vi "rvc SIM Quadcopter.vi"(7 "omega2":dbl, 9 "omega4":dbl, 10 "omega3":dbl, 11 "omega1":dbl) -> (3 "States":dbl[](array[numeric])=[0.0, 0.0, 0.0, 2.3184100418409948, 0.0, 0.0])   [LabVIEW 2013]
uses:
  <vilib>/Simulation/Implementation/Shared/SIMSCR Execution Mode.ctl
  <vilib>/Simulation/Scripting/Companion Diagram/SimConfigNode/SimParams.ctl
  <vilib>/Simulation/Scripting/Companion Diagram/SimConfigNode/_simSolvers.ctl
  <vilib>/Simulation/Param Hierarchy/Typedefs/SIMPH Param Control Actions.ctl
  <vilib>/Simulation/Implementation/Shared/SIM limit type.ctl
  <vilib>/Simulation/Implementation/Shared/NILVSim_ParamChanged.vi
  <vilib>/Simulation/Implementation/Shared/NILVSIM_BeginStep.vi
  <vilib>/Simulation/ContinuousLinear/Implementation/NILVSim Integrator new.llb/SIM Integrator Distributor (vector).vi
  <vilib>/Simulation/ContinuousLinear/Implementation/NILVSim Integrator new.llb/SIM Integrator Collector (vector).vi
  <vilib>/Simulation/Implementation/Shared/NILVSim_Manager.vi
  <vilib>/Simulation/Implementation/Shared/NILVSim_FinalizeModel.vi
  <vilib>/Simulation/Implementation/Shared/SIM Unbundle Sim Info.vi
  <vilib>/Utility/error.llb/Clear Errors.vi
  <vilib>/Simulation/Implementation/Shared/NILVSim_GetModelError.vi
  <vilib>/Simulation/Implementation/Shared/SIM SimErrorHandler.vi
  <vilib>/Simulation/Implementation/Shared/SIM Bundle Sim Info.vi
  <vilib>/Simulation/Implementation/Shared/SIMSH Read Queue.vi
  <vilib>/Simulation/Implementation/Shared/NILVSim_Initialize.vi
  <vilib>/Simulation/Utility/Implementation/NILVSim Get Time and IsAcceptedStep.vi
  <vilib>/Simulation/Scripting/Companion Diagram/SimConfigNode/SimDog.xnode
  <vilib>/Simulation/Implementation/XNodeFramework/SimXNode/SimX.xnode
  <vilib>/Simulation/ContinuousLinear/Implementation/NILVSim Integrator new.llb/SIM Integrator (vector).vi
  <vilib>/Simulation/Implementation/Shared/NI_SIM_Implementation.lvlib
panel:
  in  "drag":dbl=1.0814e-08
  in  "thrust":dbl=1.0814e-06
  out "Position States":dbl[](array[numeric])=[0.0, 0.0, 0.0, 11.592050209204974, 0.0, 0.0]
  out "Velocity States":dbl[](array[numeric])=[0.0, 0.0, 0.0, 2.3184100418409948, 0.0, 0.0]
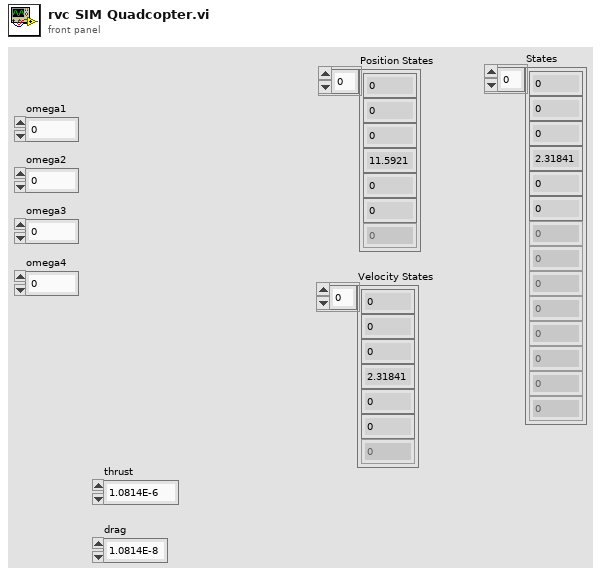
[diagram p1: front panel]
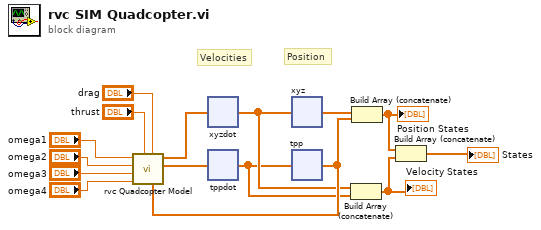
[diagram p0: block diagram]
diagram:
  # "Position"
  # "Velocities"
  n1 = call "rvc Quadcopter Model.vi"("tpp"=w7, "d"="drag", "b"="thrust", "omega4"="omega4", "omega3"="omega3", "omega2"="omega2", "omega1"="omega1") -> ("tpp_2dot 2"=w9:dbl[], "xyz_2dot"=w1:dbl[])  [unwired: 3 in]
  n2 = xnode "xyzdot"("input"=w1) -> ("output"=w6:dbl[])  [unwired: 9 in, 2 out]
  n3 = xnode "tppdot"("input"=w9) -> ("output"=w5:dbl[])  [unwired: 9 in, 2 out]
  n4 = xnode "xyz"("input"=w6) -> ("output"=w8:dbl[])  [unwired: 9 in, 2 out]
  n5 = xnode "tpp"("input"=w5) -> ("output"=w7:dbl[])  [unwired: 9 in, 2 out]
  n6 = Build Array (concatenate) ("Build Array 2")(w6, w5) -> (w4:dbl[])
  "Velocity States" <- w4
  n7 = Build Array (concatenate)(w8, w7) -> (w3:dbl[])
  "Position States" <- w3
  n8 = Build Array (concatenate) ("Build Array 3")(w3, w4) -> (→"States":dbl[])
